vi "TCP_client.vi"() -> ()   [LabVIEW 2018]
panel:
  in  "stop":bool
  out "send_Data":string
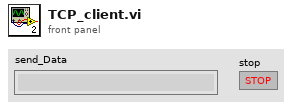
[diagram p1: front panel]
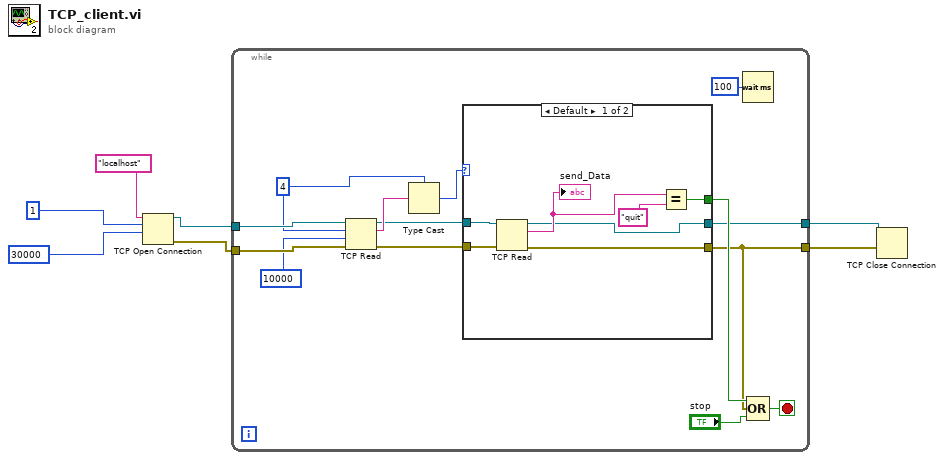
[diagram p0: block diagram]
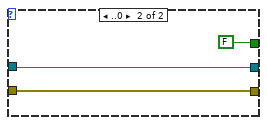
[diagram p2: hidden frame]
diagram:
  n1 = TCP Open Connection(address="localhost", remote port or service name=1, timeout ms (60000)=30000) -> (connection ID=w2:refnum<k5>, error out=w3:errorcluster)  [unwired: 2 in]
  n2 = while {
    tunnel: w2 -> [w21]
    tunnel: w3 -> [w20]
    tunnel: [w9] -> w7
    tunnel: [w8] -> w6
    stop <- w12 stop-if-true
    w17 = 4
    n3 = TCP Read(connection ID=w21, bytes to read=w17, error in (no error)=w20, 9:10000) -> (connection ID out=w15:refnum<k5>, data out=w18:string, error out=w14:errorcluster)  [unwired: 1 in]
    n4 = Type Cast(type=w17, x=w18) -> (*(type *) &x=w16:i32)
    n5 = case shown="Default" w16 {
      tunnel: w15 -> [w28 w31]
      tunnel: w14 -> [w27 w30]
      tunnel: [w24 FALSE] -> w10
      tunnel: [w23 w30] -> w9
      tunnel: [w22 w31] -> w8
      frame Default {
        n6 = TCP Read(connection ID=w28, error in (no error)=w27) -> (connection ID out=w22:refnum<k5>, data out=w26:string, error out=w23:errorcluster)  [unwired: 3 in]
        "send_Data" <- w26
        n7 = Equal?(x=w26, y="quit") -> (x = y?=w24:bool)
      }
      frame ..0 {
      }
    }
    n8 = Wait (ms)(milliseconds to wait=100) -> ()  [unwired: 1 out]
    n9 = Compound Arithmetic op=OR(w10, w9, "stop") -> (w12:bool)
  }
  n10 = TCP Close Connection(connection ID=w6, error in (no error)=w7) -> ()  [unwired: 1 in, 2 out]
